vi "set switch.vi"(8 "error in (no error)":errorcluster, 9 "state":bool, 10 "channel":dbl, 11 "Qtegra in":refnum<class "Qtegra.lvclass">) -> (0 "error out":errorcluster, 3 "Qtegra out":refnum<class "Qtegra.lvclass">)   [LabVIEW 2017, in "Qtegra.lvclass"]
uses:
  Qtegra.lvclass
  \\Mac\Home/my data/University/Lamont/Software/LabView/MSControlSuite_Code/MSControl/Classes/Instrument/instrument.lvclass
  instrument.lvclass
panel:
  out "data out":string
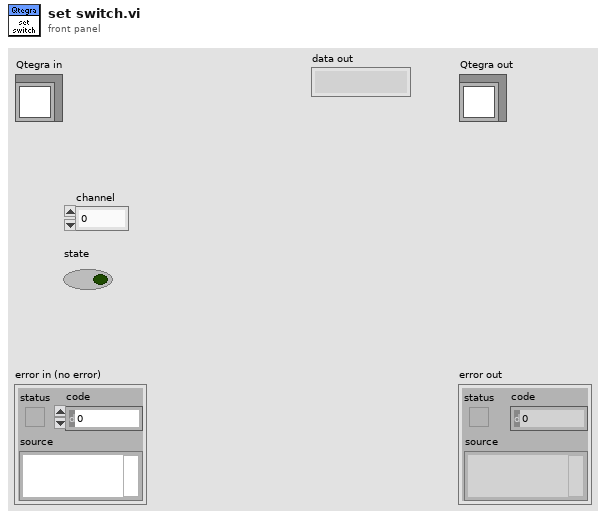
[diagram p1: front panel]
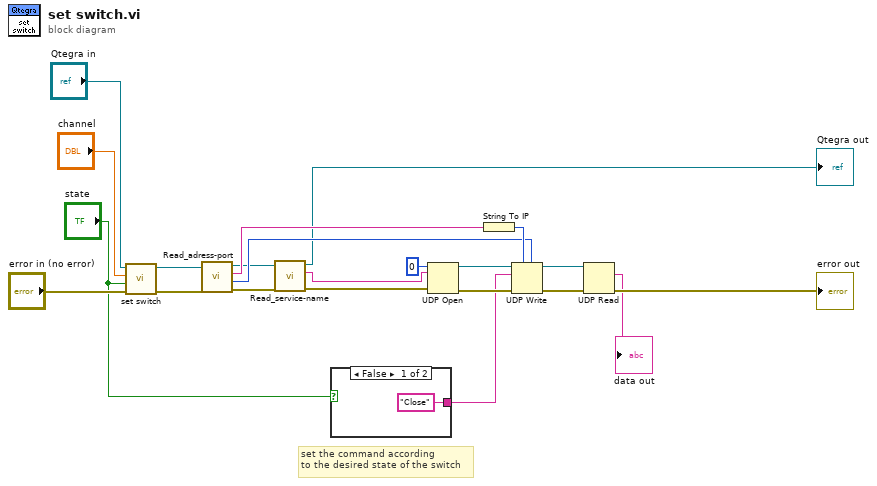
[diagram p0: block diagram]
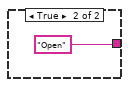
[diagram p2: hidden frame]
diagram:
  # "set the command according\nto the desired state of the switch"
  n1 = call-parent "set switch.vi"("error in (no error)"="error in (no error)", "state"="state", "channel"="channel", "instrument in"="Qtegra in") -> ("error out"=w5:errorcluster, "instrument out"=w6:refnum<class "Qtegra.lvclass">)  [unwired: 6 in]
  n2 = call "Read_adress-port.vi"("error in (no error)"=w5, "instrument in"=w6) -> ("error out"=w11:errorcluster, "port number"=w12:i32, "adress"=w19:string, "instrument out"=w10:refnum<class "Qtegra.lvclass">)  [unwired: 6 in]
  n3 = call-dynamic "Read_service-name.vi"("error in (no error)"=w11, "instrument in"=w10) -> ("error out"=w9:errorcluster, "service name"=w8:string, "instrument out"=→"Qtegra out":refnum<class "Qtegra.lvclass">)  [unwired: 7 in]
  n4 = case shown="False" "state" {
    tunnel: ["Close" "Open"] -> w7
    frame False {
    }
    frame True {
    }
  }
  n5 = UDP Open(8:w9, 10:w8, 11:u16 0 ("port")) -> (port=w15:refnum<k16>, 0:w16:errorcluster)  [unwired: 2 in, 1 out]
  n6 = String To IP(1:w19) -> (0:w18:u32)
  n7 = UDP Write(address=w18, port or service name=w12, connection ID=w15, data in=w7, 8:w16) -> (error out=w13:errorcluster, 3:w14:refnum<k16>)  [unwired: 1 in]
  n8 = UDP Read(connection ID=w14, 8:w13) -> (data out=→"data out":string, error out=→"error out":errorcluster)  [unwired: 2 in, 3 out]
